vi "ToolingPinAnalysis.vi"() -> ()   [LabVIEW 2016]
uses:
  <vilib>/vision/Measure.llb/Straight Edge Options.ctl
  <vilib>/vision/Measure.llb/Straight Edge Process.ctl
  <vilib>/vision/Measure.llb/Edge Options.ctl
  <vilib>/vision/Measure.llb/Edge Polarity.ctl
  <vilib>/Analysis/6fits.llb/Curve Fitting Criteria.ctl
  <vilib>/Utility/file.llb/Write Delimited Spreadsheet (DBL).vi
  <vilib>/regexp/Match Regular Expression.xnode
  <vilib>/Analysis/NI_AALPro.lvlib
panel:
  in  "Number of images each":i32=10
  in  "Number of pins":i32=5
  out "y errors (mm)":dbl[](array[numeric])
  out "x errors (mm)":dbl[](array[numeric])
  in  "stop":bool
  out "Bottom Residue":dbl
  out "Top residue":dbl
  in  "x values for fit line on plot":dbl[](array[numeric])=[-700.0, -300.0, 100.0, 500.0, 700.0]
  out "Bottom intercept":dbl
  out "Bottom slope":dbl
  out "Top intercept":dbl
  in  "method":T1 items=["Least Square", "Least Absolute Residual", "Bisquare"]
  out "Top slope":dbl
  out "Each point on located edges":T2(graph)
  out "Coordinate array for image capture":dbl[][](array[numeric])
  in  "Coordinate file for image capture":path=path "E:/XYZstage+Camera_CollectedImages/12-16-2016/noStaveMount/toolingpinsCoordinates-captured.csv"
  out "Review":bool
  out "Search running?":bool
  in  "Options: Bottom Edge Search":T5={"Search Direction"=3, "Edge Options"={"Edge Polarity"=2, "Kernel Size"=9, "Width"=3, "Minimum Edge Strength"=17.0, "Interpolation Type"=enum."Bilinear Fixed", "Data Processing Method"=enum."Average"}, "Show Search Area"=TRUE, "Show Search Lines"=TRUE, "Show Edges Found"=TRUE, "Show Result"=TRUE, "Search Area Color"=65280, "Search Lines Color"=255, "Edge Locations Color"=16776960, "Result Color"=16711680, "Overlay Group Name"=""} {"Search Direction" items=["Left to Right", "Right to Left", "Top to Bottom", "Bottom to Top"]; "Edge Options"."Edge Polarity" items=["All Edges", "Rising Edges", "Falling Edges"]; "Edge Options"."Minimum Edge Strength" format="%.2f"; "Edge Options"."Width" step=2; "Edge Options"."Kernel Size" step=2}
  in  "Options: Top Edge Search":T5={"Search Direction"=2, "Edge Options"={"Edge Polarity"=0, "Kernel Size"=5, "Width"=3, "Minimum Edge Strength"=16.0, "Interpolation Type"=enum."Bilinear Fixed", "Data Processing Method"=enum."Average"}, "Show Search Area"=TRUE, "Show Search Lines"=TRUE, "Show Edges Found"=TRUE, "Show Result"=TRUE, "Search Area Color"=65280, "Search Lines Color"=255, "Edge Locations Color"=16776960, "Result Color"=16711680, "Overlay Group Name"=""} {"Search Direction" items=["Left to Right", "Right to Left", "Top to Bottom", "Bottom to Top"]; "Edge Options"."Edge Polarity" items=["All Edges", "Rising Edges", "Falling Edges"]; "Edge Options"."Minimum Edge Strength" format="%.2f"; "Edge Options"."Width" step=2; "Edge Options"."Kernel Size" step=2}
  in  "Fit Options":T6={"Number of Lines"=1, "Type"=enum."First Edge Rake", "Min. Score"=10.0, "Max. Score"=1000.0, "Orientation"=0.0, "Angle Range"=45.0, "Angle Tolerance"=1.0, "Step Size"=196, "Min. SNR (db)"=0.0, "Min. Points (%)"=25.0, "Hough Iterations"=5} {"Min. Points (%)" min=0.0 max=100.0; "Min. SNR (db)" min=0.0; "Max. Score" min=0.0 max=1024.0; "Min. Score" min=0.0 max=1024.0 step=1.0}
  in  "Stop and delete":bool
  out "Images Array":T8[](array[plugin-control])
  in  "error in":errorcluster
  out "error out":errorcluster
  out "Filenames Array":string[](array[string])
  in  "Naming Convention":string="*.png"
  in  "Images Directory":path=path "E:/XYZstage+Camera_CollectedImages/12-16-2016/noStaveMount/toolingpins_images"
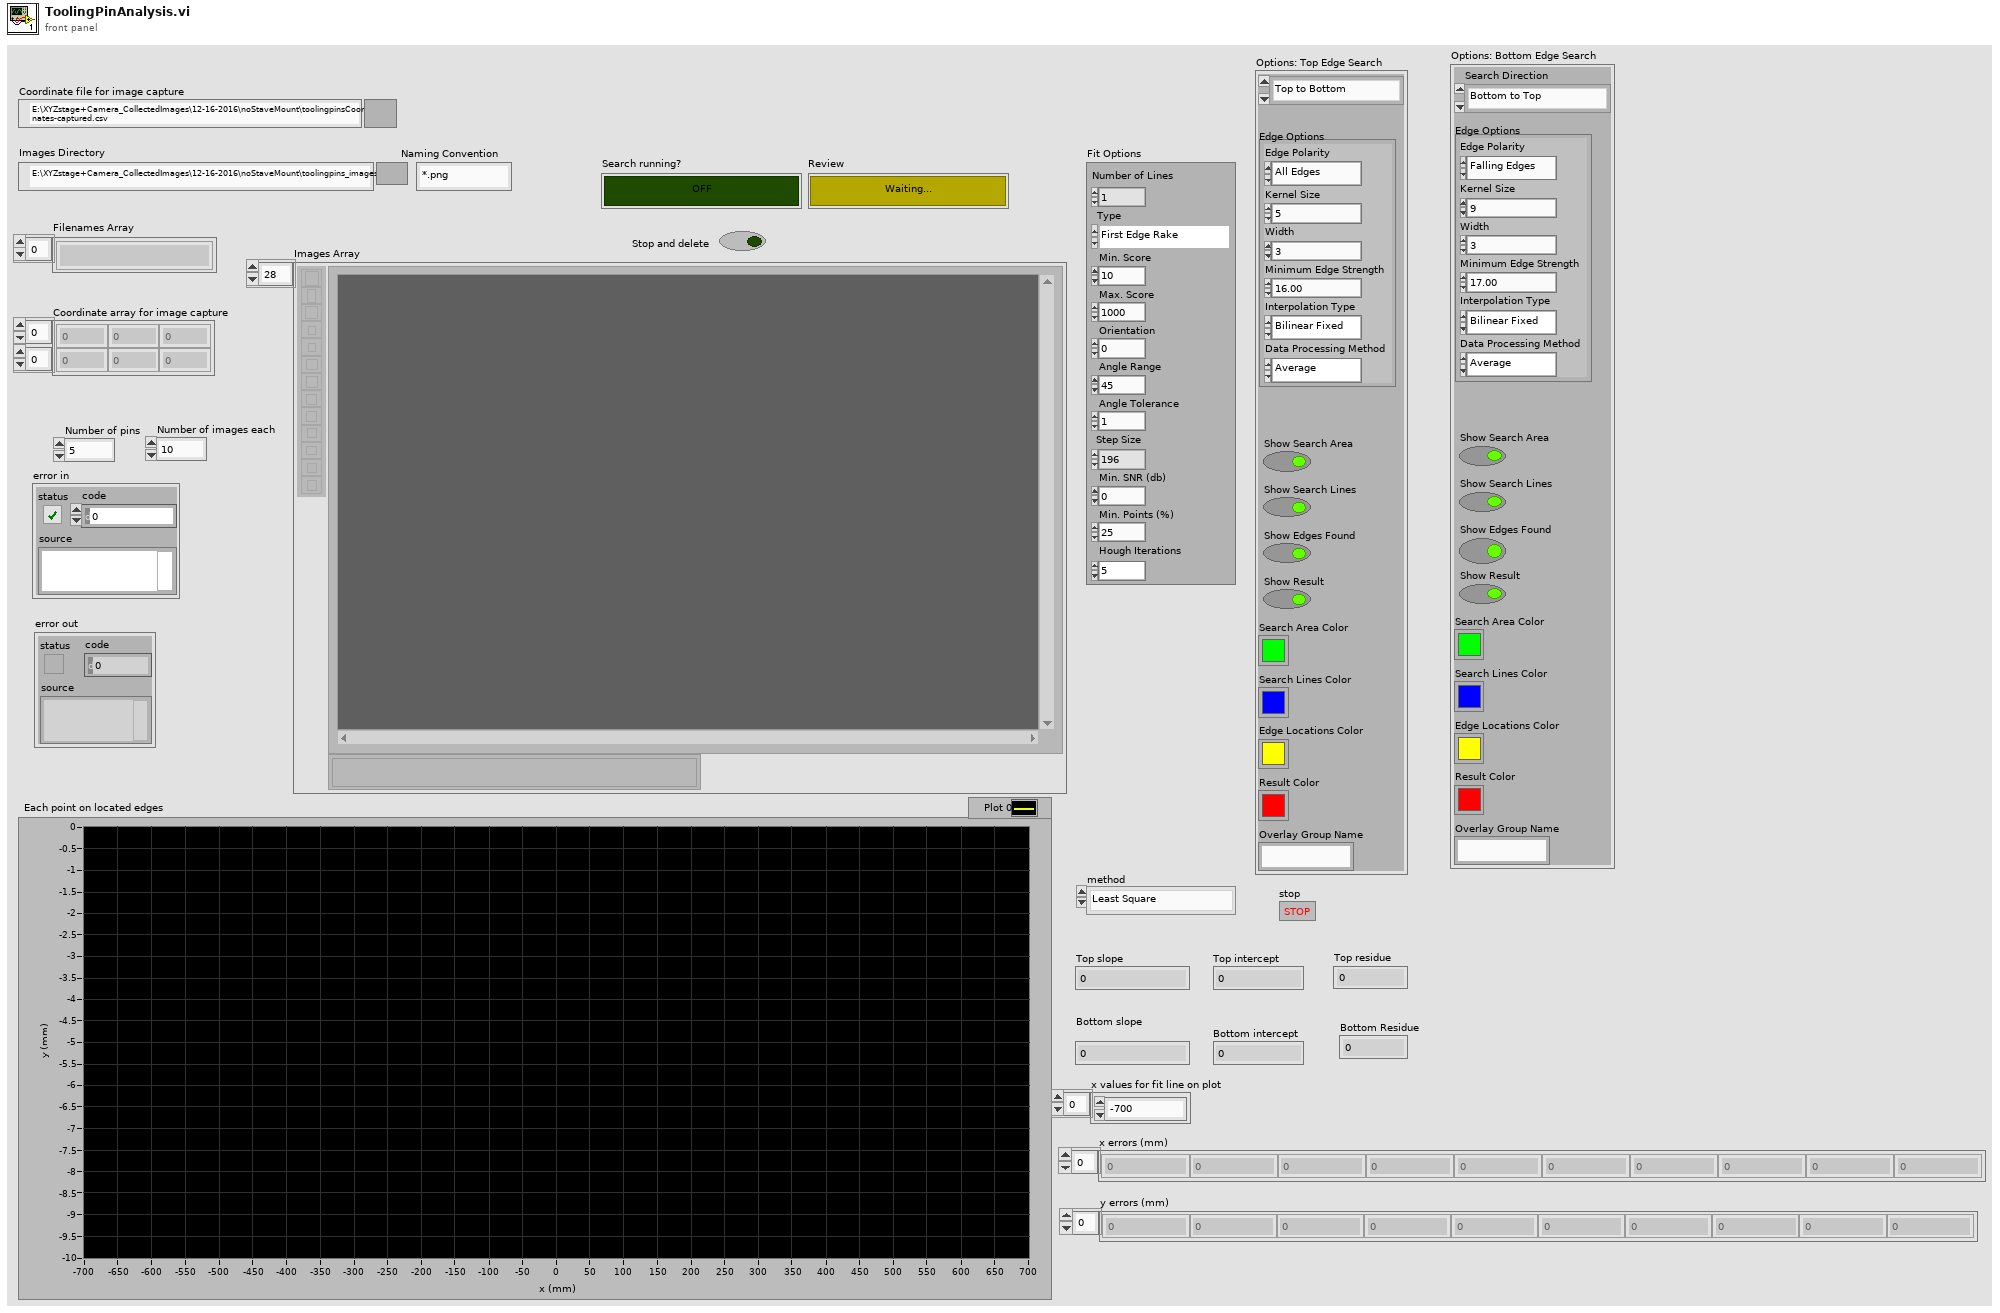
[diagram p1: front panel]
types:
  T1 = typedef "NI_AALPro.lvlib/Curve Fitting Criteria.ctl" = u16
  T2 = cluster{"Top averages":dbl[], "Best Linear Fit":dbl[]}[]
  T3 = typedef "Edge Options.ctl" = cluster{"Edge Polarity":T4, "Kernel Size":u32, "Width":u32, "Minimum Edge Strength":sgl, "Interpolation Type":enum32{"Zero Order", "Bilinear", "Quadratic", "Cubic", "Bilinear Fixed"}, "Data Processing Method":enum32{"Average", "Median"}}
  T4 = typedef "Edge Polarity.ctl" = u32
  T5 = cluster{"Search Direction":u32, "Edge Options":T3, "Show Search Area":bool, "Show Search Lines":bool, "Show Edges Found":bool, "Show Result":bool, "Search Area Color":u32, "Search Lines Color":u32, "Edge Locations Color":u32, "Result Color":u32, "Overlay Group Name":string}
  T6 = typedef "Straight Edge Options.ctl" = cluster{"Number of Lines":i32, "Type":T7, "Min. Score":dbl, "Max. Score":dbl, "Orientation":dbl, "Angle Range":dbl, "Angle Tolerance":dbl, "Step Size":u32, "Min. SNR (db)":dbl, "Min. Points (%)":dbl, "Hough Iterations":i32}
  T7 = typedef "Straight Edge Process.ctl" = enum32{"First Edge Rake", "Best Edge Rake", "Hough Edge Rake", "First Edge Projection", "Best Edge Projection"}
  T8 = typedef "IMAQ Image.ctl" = refnum<image>
  T9 = enum16{"cm", "mm", "pixels [mm/pix]", "pixels [um/pix]"}
  T10 = cluster{"Top Averages":dbl[], "Top Averages":dbl[]}
  T11 = cluster{"x values for fit line on plot":dbl[], "Array":dbl[]}
  T12 = cluster{"x values for fit line on plot":dbl[], "Array":dbl[]}[]
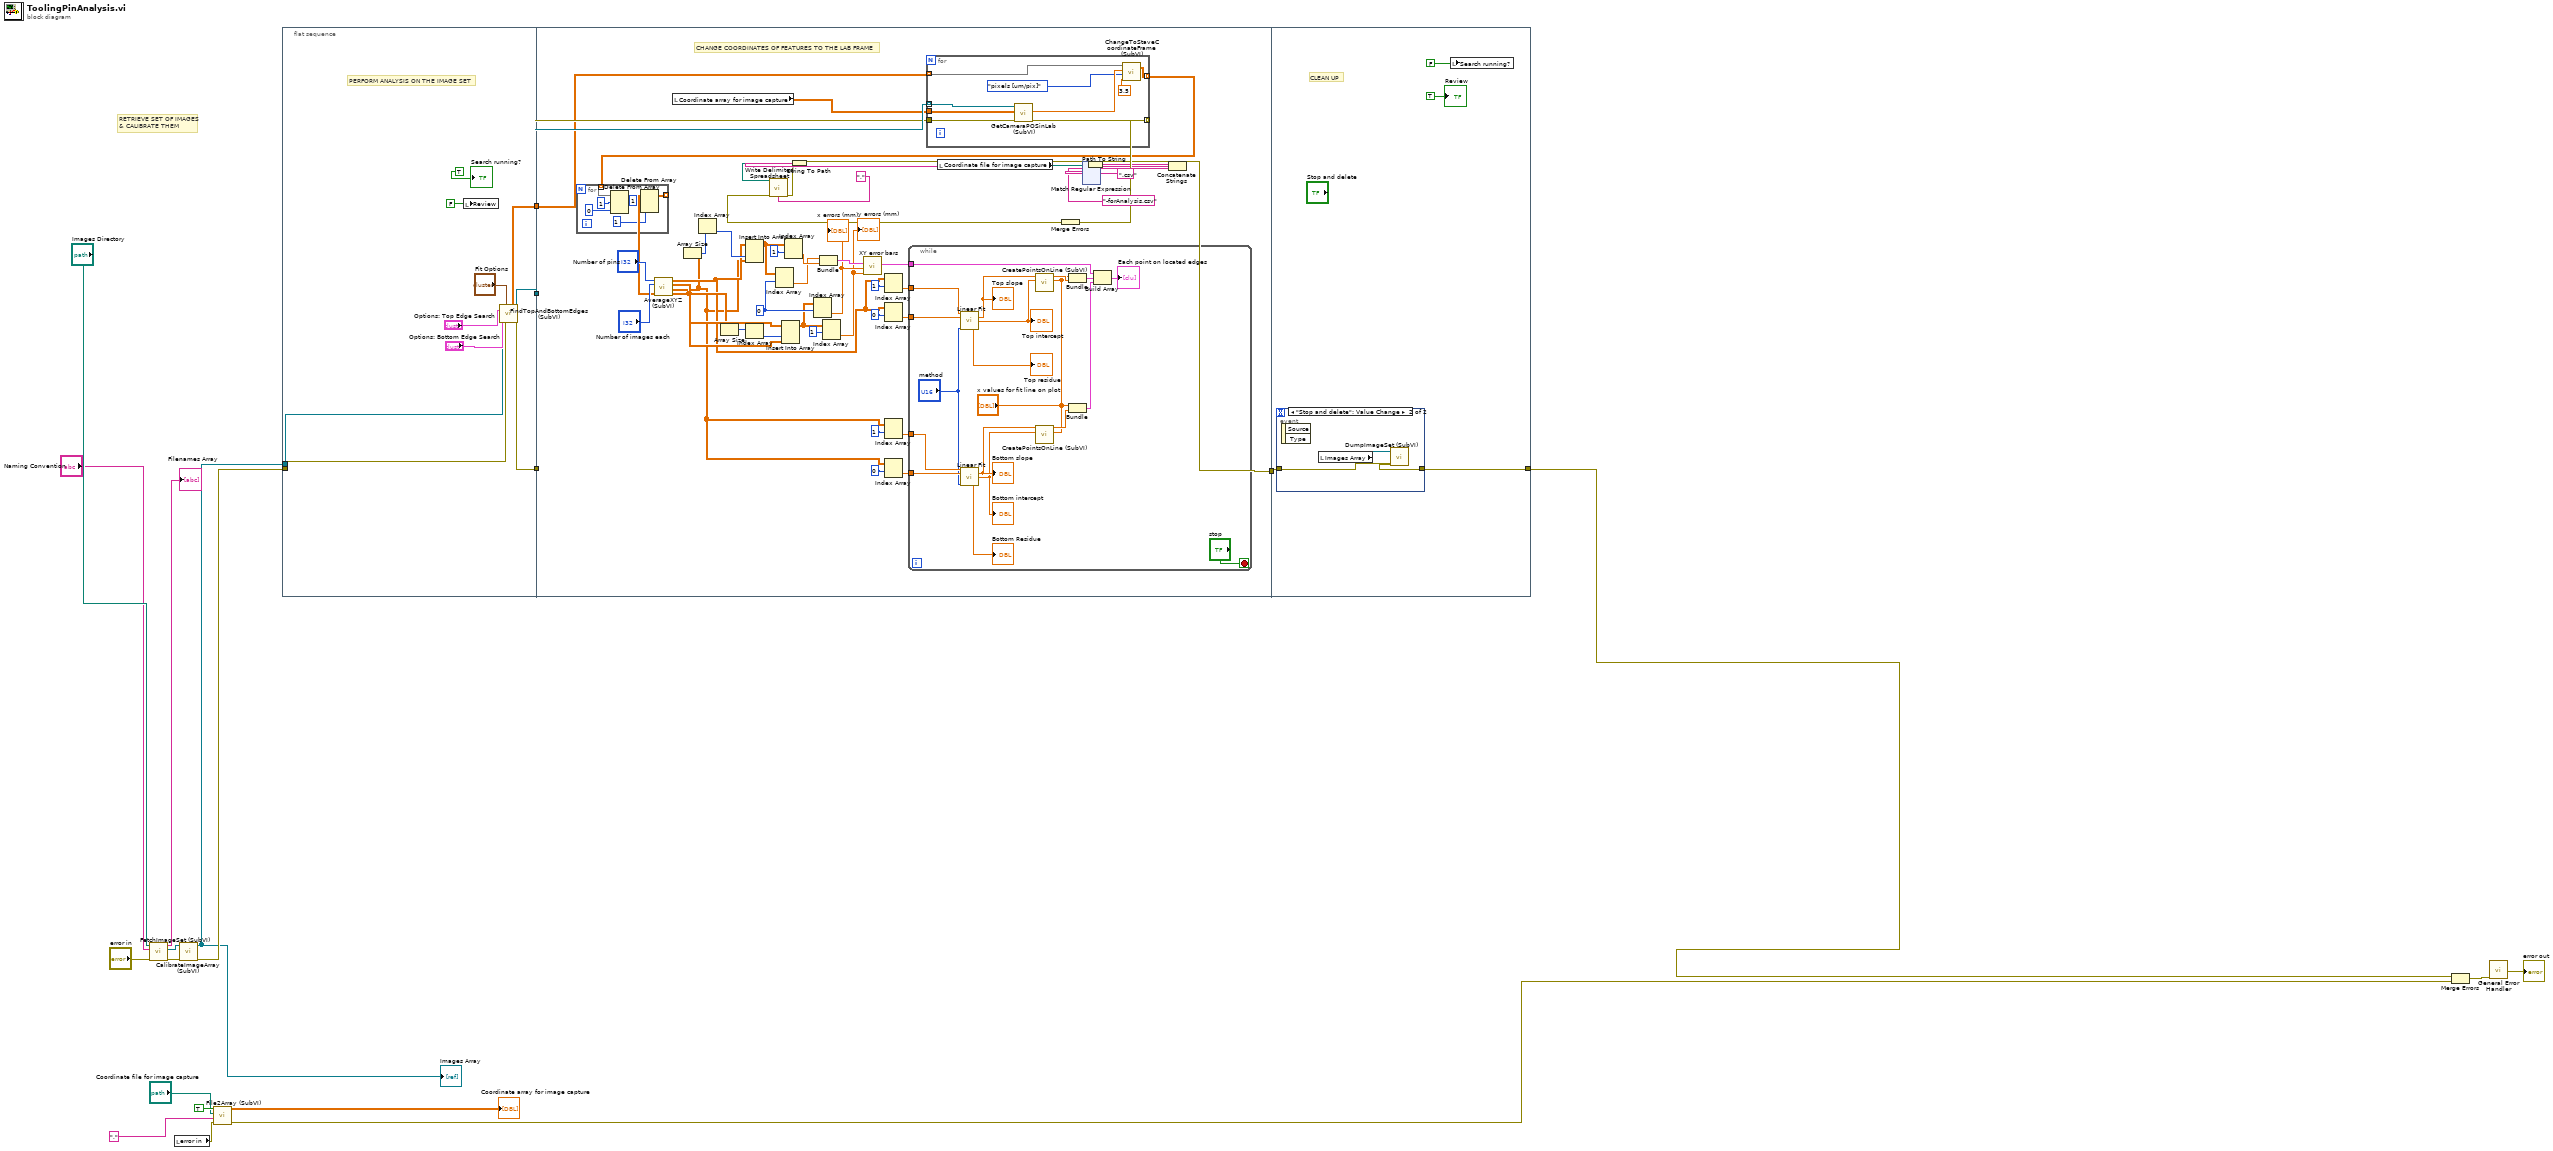
[diagram p0: block diagram]
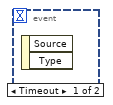
[diagram p2: hidden frame]
diagram:
  # "RETRIEVE SET OF IMAGES\n& CALIBRATE THEM"
  n1 = call "FetchImageSet (SubVI).vi"("error in (no error)"="error in", "Naming Convention"="Naming Convention", "Images Directory"="Images Directory") -> ("error out"=w17:errorcluster, "Image Array"=w18:T8[], "Filenames Array"=→"Filenames Array":string[])  [unwired: 6 in]
  n2 = local read "error in"() -> (w7:errorcluster)
  n3 = call "CalibrateImageArray (SubVI).vi"("error in (no error)"=w17, "Image Array"=w18) -> ("error out"=w14:errorcluster, "Calibrated Image Array"=w13:T8[])  [unwired: 7 in]
  "Images Array" <- w13
  n4 = call "File2Array (SubVI).vi"("error in (no error) in"=w7, "File delimiter"=",", "Source array file"="Coordinate file for image capture", "Load array from file?"=TRUE) -> ("error in (no error) out"=w5:errorcluster, "Loaded array"=→"Coordinate array for image capture":dbl[][])  [unwired: 6 in]
  n5 = flat-sequence {
    tunnel: w14 -> [w31]
    tunnel: w13 -> [w22]
    tunnel: [w30] -> w12
    tunnel: [w29] -> w11
    tunnel: [w23] -> w3
    tunnel: w12 -> [w76]
    tunnel: w11 -> [w77]
    tunnel: w3 -> [w74]
    tunnel: [w63] -> w2
    tunnel: [w228] -> w6
    tunnel: w2 -> [w227]
    frame #0 {
      # "PERFORM ANALYSIS ON THE IMAGE SET"
      n6 = local write "Review"(FALSE ("Review")) -> ()
      n7 = call "FindTopAndBottomEdges (SubVI).vi"("Calibrated Image Array"=w22, "Fit Options"="Fit Options", "Options: Top Edge Search"="Options: Top Edge Search", "Options: Bottom Edge Search"="Options: Bottom Edge Search", "error in (no error)"=w31) -> ("Analyzed Image Array"=w29:T8[], "Array of Edge Endpoint Arrays"=w23:sgl[][][], "error out"=w30:errorcluster)  [unwired: 6 in, 2 out]
      "Search running?" <- TRUE ("Search running?")
    }
    frame #1 {
      w61 = 0 ("index (row)")
      # "CHANGE COORDINATES OF FEATURES TO THE LAB FRAME"
      n8 = local read "Coordinate array for image capture"() -> (w75:dbl[][])
      n9 = for {
        tunnel: w77 -> [w226] mode=indexing
        tunnel: w76 -> [w225]
        tunnel: w75 -> [w224]
        tunnel: w74 -> [w222] mode=indexing
        tunnel: [w219] -> w73 mode=indexing
        tunnel: [w218] -> w33 mode=indexing
        n10 = call "GetCameraPOSinLab (SubVI).vi"("error in (no error)"=w225, "Loaded array"=w224, "Refnum in"=w226) -> ("error out"=w219:errorcluster, "Image coordinates in lab frame"=w223:dbl[])  [unwired: 6 in, 1 out]
        n11 = call "ChangeToStaveCoordinateFrame (SubVI).vi"("Loaded array (image frame)"=w222, "Image Origin in XYZ Stage Coords [mm]"=w223, "Units"=T9."pixels [um/pix]", "Pixel resolution"=3.5) -> ("Array (stage frame, mm)"=w218:dbl[][])  [unwired: 2 in]
      }
      n12 = for {
        tunnel: w33 -> [w84] mode=indexing
        tunnel: [w80] -> w32 mode=indexing
        n13 = Delete From Array(array=w84, length=1, index (row)=0) -> (array with subset deleted=w81:dbl[][])  [unwired: 1 in, 1 out]
        n14 = Delete From Array(array=w81, length=1, index (row)=1) -> (array with subset deleted=w80:dbl[][])  [unwired: 1 in, 1 out]
      }
      n15 = call "AverageXYZ (SubVI).vi"("array"=w32, "Number of images each"="Number of images each", "Number of pins"="Number of pins") -> ("Bottom uncertainty"=w54:dbl[][], "Bottom averages"=w39:dbl[][], "Top uncertainty"=w57:dbl[][], "Top Averages"=w44:dbl[][])  [unwired: 5 in]
      n16 = Array Size(array=w39) -> (size(s)=w60:i32[])
      n17 = Index Array(array=w60) -> (element=w59:i32)  [unwired: 1 in]
      n18 = Array Size(array=w54) -> (size(s)=w55:i32[])
      n19 = Insert Into Array(array=w44, index (col)=w59, new element=w39) -> (w58:dbl[][])  [unwired: 1 in]
      n20 = Index Array(array=w55) -> (element=w56:i32)  [unwired: 1 in]
      n21 = Index Array(array=w58, index (row)=w61) -> (element=w38:dbl[])  [unwired: 1 in]
      n22 = Insert Into Array(array=w57, index (col)=w56, new element=w54) -> (w52:dbl[][])  [unwired: 1 in]
      n23 = Index Array(array=w58, index (row)=1) -> (element=w49:dbl[])  [unwired: 1 in]
      n24 = Index Array(array=w52, index (row)=w61) -> (element=w51:dbl[])  [unwired: 1 in]
      "x errors (mm)" <- w51
      n25 = Bundle("Top Averages"=w38, "Top Averages"=w49) -> (w53:T10)  [unwired: 1 in]
      n26 = Index Array(array=w52, index (row)=1) -> (element=w50:dbl[])  [unwired: 1 in]
      "y errors (mm)" <- w50
      n27 = call "XY error bars.vi"("XY plot"=w53, "Xerror"=w51, "Yerror"=w50) -> ("X+Y error bars"=w37:cluster{dbl[], dbl[]})  [unwired: 5 in, 2 out]
      n28 = Index Array(array=w44, index (row)=1) -> (element=w46:dbl[])  [unwired: 1 in]
      n29 = Index Array(array=w44, index (row)=0) -> (element=w45:dbl[])  [unwired: 1 in]
      n30 = Index Array(array=w39, index (row)=1) -> (element=w41:dbl[])  [unwired: 1 in]
      n31 = Index Array(array=w39, index (row)=0) -> (element=w40:dbl[])  [unwired: 1 in]
      n32 = while {
        tunnel: w46 -> [w103]
        tunnel: w45 -> [w102]
        tunnel: w41 -> [w101]
        tunnel: w40 -> [w100]
        tunnel: w37 -> [w99]
        stop <- "stop" stop-if-true
        n33 = call <vilib>:"Linear Fit.vi"("Y"=w103, "X"=w102, "method"="method") -> ("slope"=w98:dbl, "intercept"=w97:dbl, "residue"=→"Top residue":dbl)  [unwired: 8 in, 2 out]
        "Top slope" <- w98
        "Top intercept" <- w97
        n34 = call <vilib>:"Linear Fit.vi"("Y"=w101, "X"=w100, "method"="method") -> ("slope"=w94:dbl, "intercept"=w88:dbl, "residue"=→"Bottom Residue":dbl)  [unwired: 8 in, 2 out]
        "Bottom slope" <- w94
        "Bottom intercept" <- w88
        n35 = call "CreatePointsOnLine (SubVI).vi"("x values for fit line on plot"="x values for fit line on plot", "intercept"=w97, "slope"=w98) -> ("Array"=w96:dbl[])  [unwired: 8 in]
        n36 = call "CreatePointsOnLine (SubVI).vi"("x values for fit line on plot"="x values for fit line on plot", "intercept"=w88, "slope"=w94) -> ("Array"=w95:dbl[])  [unwired: 8 in]
        n37 = Bundle("x values for fit line on plot"="x values for fit line on plot", "Array"=w96) -> (w92:T11)  [unwired: 1 in]
        n38 = Bundle("x values for fit line on plot"="x values for fit line on plot", "Array"=w95) -> (w93:T11)  [unwired: 1 in]
        n39 = Build Array(w99, w92, w93) -> (→"Each point on located edges":T12)
      }
      n40 = local read "Coordinate file for image capture"() -> (w72:path)
      n41 = Merge Errors(w73) -> (w64:errorcluster)
      n42 = Path To String(path=w72) -> (string=w70:string)
      n43 = xnode "Match Regular Expression"("input string"=w70, "regular expression"=".csv") -> ("before match"=w68:string)  [unwired: 4 in, 4 out]
      n44 = Concatenate Strings(w68, "-forAnalysis.csv" ("name or relative path")) -> (w67:string)
      n45 = String To Path(string=w67) -> (path=w65:path)
      n46 = call-poly <vilib>:"Write Delimited Spreadsheet.vi"("file path (dialog if empty)"=w65, "error in (no error)"=w64, "delimiter (\\t)"="," ("delimiter (\\t)")) -> ("error out"=w63:errorcluster)  [unwired: 11 in, 1 out]
    }
    frame #2 {
      # "CLEAN UP"
      n47 = event shown="[1] \"Stop and delete\": Value Change" {
        selector: _ -> [_ _]
        dyn-events: _ -> [_ _]
        timeout: _ -> [_ _]
        tunnel: [_ w233] -> w228
        tunnel: w227 -> [_ w232]
        event Timeout {
          n48 = event-data() -> ()  [unwired: 1 in, 2 out]
        }
        event "Stop and delete": Value Change {
          n49 = event-data() -> ()  [unwired: 1 in, 2 out]
          n50 = local read "Images Array"() -> (w231:T8[])
          n51 = call "DumpImageSet (SubVI).vi"("error in (no error)"=w232, "Calibrated Image Array"=w231) -> ("error out"=w233:errorcluster)  [unwired: 6 in]
        }
      }
      n52 = local write "Search running?"(FALSE ("Search running?")) -> ()
      "Review" <- TRUE ("Review")
    }
  }
  n53 = Merge Errors(w6, w5) -> (w4:errorcluster)
  n54 = call <vilib>:"General Error Handler.vi"("error in (no error)"=w4) -> ("error out"=→"error out":errorcluster)  [unwired: 10 in, 4 out]
